vi "Flat Field Estimation.vi"() -> ()   [LabVIEW 2018]
doc: "This example illustrates flat field estimation algorithm. This algorithm estimates the flat field image by surface fitting the background region of the image. Flat field estimation follows two step process. It calculates the background image by using local thresholding methods or surface fitting mathematical model. Once the background image is calculated, surface fit is applied on background image to estimate the flat field image."
uses:
  <vilib>/vision/Process.llb/Background Estimation Options.ctl
  <vilib>/vision/Process.llb/Surface Fit Options.ctl
  <vilib>/vision/NI_Vision_Development_Module.lvlib
panel:
  in  "path":path
  in  "Show Estimated Image?":bool
  in  "Stop":bool
  out "Histograph":T1(graph)
  out "Corrected/Estimated Image":T2(plugin-control)
  out "Part Image":T2(plugin-control)
  in  "Select Image":i32(slide) min=0 max=5 step=1 scale=0.0..3.0
  # "Overview: Demonstrates how to use IMAQ Estimate Flat Field Model to estimate the flat filed image and correct the non uniform intensity using IMAQ Flat Field Correction.\nInstructions:\n1. Run the VI.\n2. Choose images using Select Image control.\n3. Observe the Histograph to understand the impact of correction.\n4. Enable Show Estimated Image boolean to display the estimated flat filed image."
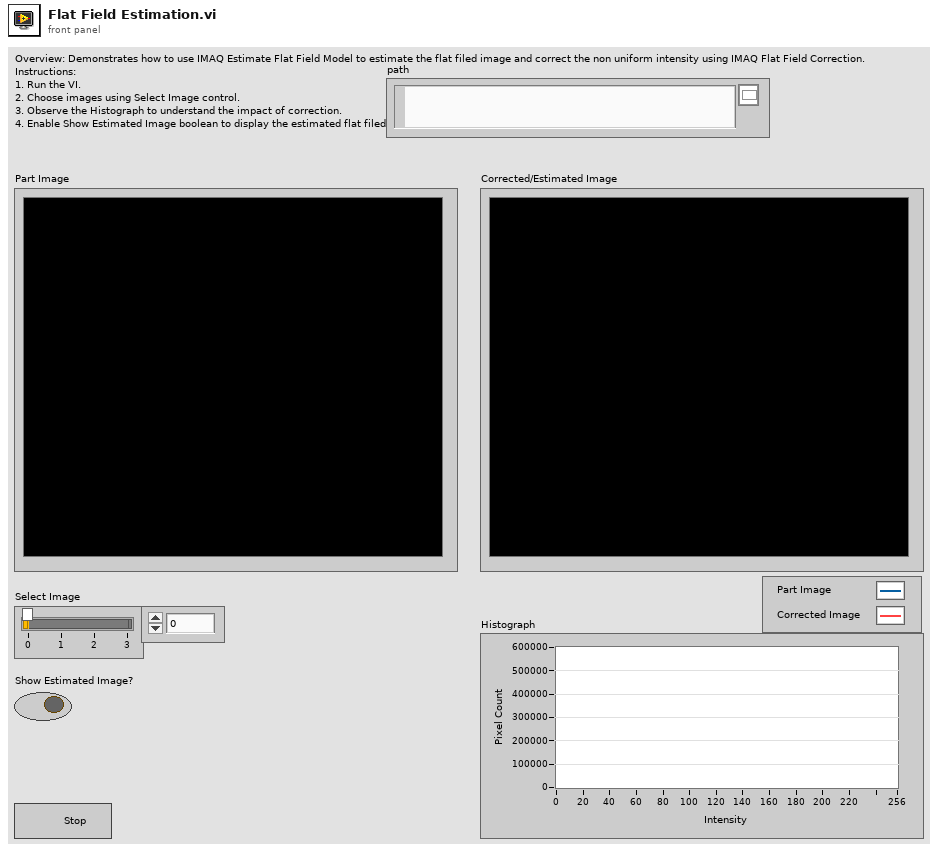
[diagram p1: front panel]
types:
  T1 = cluster{"Starting Value":sgl, "Incremental Value":sgl, "Histogram":u32[]}[]
  T2 = typedef "IMAQ Image.ctl" = refnum<image>
  T3 = typedef "Image Type" = u32
  T4 = cluster{"Line Scan Image?":bool, "Correction Factor":sgl}
  T5 = typedef "Surface Fit Options.ctl" = cluster{"Model":i32, "Sampling Grid Size":cluster{"SizeX":i32, "SizeY":i32}, "Polynomial Degree":i32}
  T6 = typedef "Background Estimation Options.ctl" = cluster{"Estimate Background?":bool, "Method":i32, "Polynomial Degree":i32, "Window Size (32x32)":cluster{"SizeX":i32, "SizeY":i32}, "Niblack Deviation Factor (0.2)":dbl}
  T7 = cluster{"Starting Value":sgl, "Incremental Value":sgl, "Histogram":u32[]}
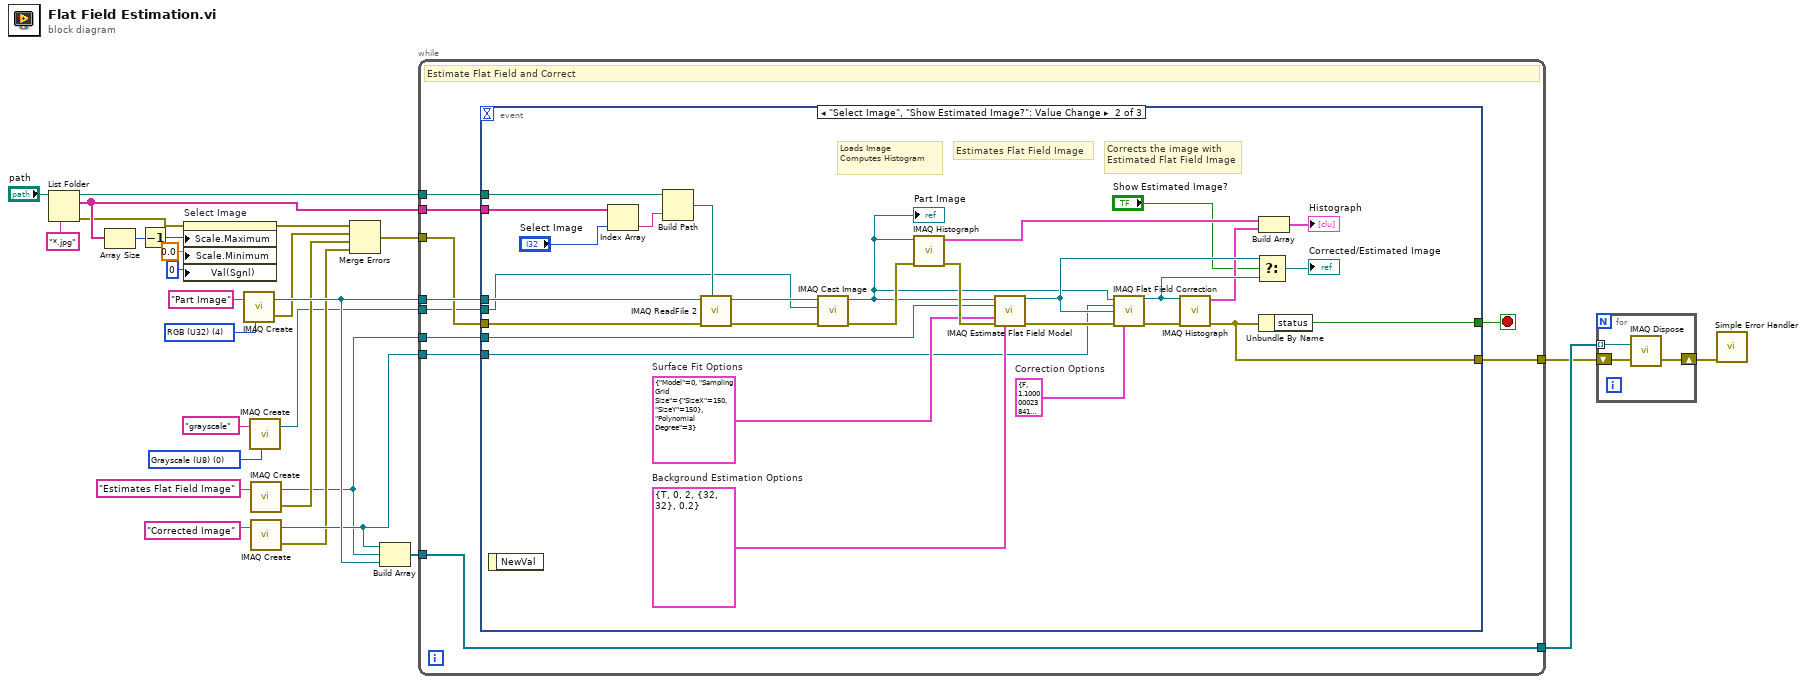
[diagram p0: block diagram]
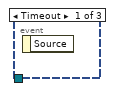
[diagram p2: hidden frame]
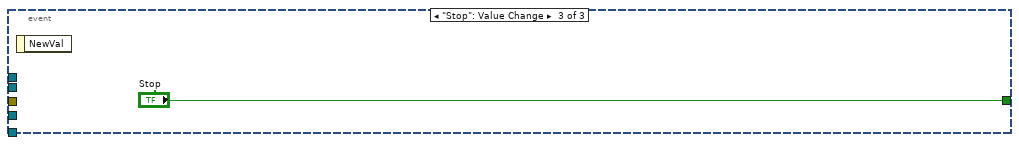
[diagram p3: hidden frame]
diagram:
  w1 = T3 0 items=["Grayscale (U8)", "Grayscale (I16)", "Grayscale (SGL)", "Complex (CSG)", "RGB (U32)", "HSL (U32)", "RGB (U64)", "Grayscale (U16)"] ("Image Type")
  w4 = T3 4 items=["Grayscale (U8)", "Grayscale (I16)", "Grayscale (SGL)", "Complex (CSG)", "RGB (U32)", "HSL (U32)", "RGB (U64)", "Grayscale (U16)"] ("Image Type")
  n1 = List Folder(path="path", pattern="*.jpg") -> (path out=w27:path, filenames=w28:string[], error out=w12:errorcluster)  [unwired: 1 in, 2 out]
  n2 = Array Size(array=w28) -> (size(s)=w24:i32)
  n3 = Decrement(x=w24) -> (x-1=w23:i32)
  n4 = property on="Select Image" class="Slide (strict)"(error in=w12, "Scale.Maximum"=w23, "Scale.Minimum"=0.0 ("Scale.Range:Minimum"), "Val(Sgnl)"=0 ("Value (Signaling)")) -> (error out=w11:errorcluster)  [unwired: 1 in, 1 out]
  n5 = call "IMAQ Create"("Image Name"="Part Image", "Image Type"=w4) -> ("New Image"=w19:T2, "error out"=w17:errorcluster)  [unwired: 3 in]
  n6 = call "IMAQ Create"("Image Name"="grayscale", "Image Type"=w1) -> ("New Image"=w2:T2)  [unwired: 3 in, 1 out]
  n7 = call "IMAQ Create"("Image Name"="Estimates Flat Field Image") -> ("New Image"=w14:T2, "error out"=w16:errorcluster)  [unwired: 4 in]
  n8 = call "IMAQ Create"("Image Name"="Corrected Image") -> ("New Image"=w18:T2, "error out"=w15:errorcluster)  [unwired: 4 in]
  n9 = Merge Errors(w11, w17, w16, w15) -> (w8:errorcluster)
  n10 = Build Array(w18, w14, w19) -> (w10:T2[])
  n11 = while {
    tunnel: w28 -> [w33]
    tunnel: w27 -> [w34]
    tunnel: w19 -> [w38]
    tunnel: w18 -> [w36]
    tunnel: w14 -> [w37]
    tunnel: [w32] -> w9
    tunnel: w10 -> [w32]
    tunnel: w8 -> [w31]
    tunnel: [w30] -> w6
    tunnel: w2 -> [w29]
    stop <- w35 stop-if-true
    # "Estimate Flat Field and Correct"
    n12 = event shown="[1] \"Select Image\", \"Show Estimated Image?\": Value Change" {
      selector: _ -> [_ _ _]
      dyn-events: _ -> [_ _ _]
      timeout: _ -> [_ _ _]
      tunnel: w38 -> [_ w43 _]
      tunnel: w37 -> [_ w53 _]
      tunnel: w36 -> [_ w52 _]
      tunnel: [_ w51 "Stop"] -> w35
      tunnel: w34 -> [_ w50 _]
      tunnel: w33 -> [_ w49 _]
      tunnel: w31 -> [_ w45 _]
      tunnel: [_ w44 _] -> w30
      tunnel: w29 -> [_ w39 _]
      event Timeout {
        n13 = event-data() -> ()  [unwired: 1 in, 1 out]
      }
      event "Select Image", "Show Estimated Image?": Value Change {
        w60 = T4 {"Line Scan Image?"=FALSE, "Correction Factor"=1.1}  # Correction Options
        w54 = T5 {"Model"=0, "Sampling Grid Size"={"SizeX"=150, "SizeY"=150}, "Polynomial Degree"=3}  # Surface Fit Options
        w55 = T6 {"Estimate Background?"=TRUE, "Method"=0, "Polynomial Degree"=2, "Window Size (32x32)"={"SizeX"=32, "SizeY"=32}, "Niblack Deviation Factor (0.2)"=0.2}  # Background Estimation Options
        # "Corrects the image with \nEstimated Flat Field Image"
        # "Estimates Flat Field Image"
        # "Loads Image \nComputes Histogram"
        n14 = event-data() -> ()  [unwired: 1 in, 1 out]
        n15 = Index Array(array=w49, index="Select Image") -> (element=w47:string)
        n16 = Build Path(base path=w50, name or relative path=w47) -> (appended path=w46:path)
        n17 = call "IMAQ ReadFile 2"("File Path"=w46, "error in (no error)"=w45, "Image"=w43) -> ("error out"=w56:errorcluster, "Image Out"=w41:T2)  [unwired: 4 in, 3 out]
        n18 = call "IMAQ Cast Image"("error in (no error)"=w56, "Image Dst"=w39, "Image Src"=w41) -> ("error out"=w42:errorcluster, "Image Dst Out"=w40:T2)  [unwired: 7 in]
        "Part Image" <- w40
        n19 = call "IMAQ Histograph"("error in (no error)"=w42, "Image"=w40) -> ("error out"=w57:errorcluster, "Histogram Graph"=w64:T7)  [unwired: 6 in, 2 out]
        n20 = call "IMAQ Estimate Flat Field Model"("Image Src"=w40, "Image Dst"=w53, "Surface Fit Options"=w54, "error in (no error)"=w57, "Background Estimation Options"=w55) -> ("Flat Field Image Out"=w66:T2, "error out"=w58:errorcluster)  [unwired: 9 in]
        n21 = call "IMAQ Flat Field Correction"("Image Src"=w40, "Image Dst"=w52, "Flat Field Image"=w66, "error in (no error)"=w58, "Correction Options"=w60) -> ("Corrected Image"=w67:T2, "error out"=w59:errorcluster)  [unwired: 8 in, 1 out]
        n22 = call "IMAQ Histograph"("error in (no error)"=w59, "Image"=w67) -> ("error out"=w44:errorcluster, "Histogram Graph"=w63:T7)  [unwired: 6 in, 2 out]
        n23 = Select(t=w66, s="Show Estimated Image?", f=w67) -> (s? t:f=→"Corrected/Estimated Image":T2)
        n24 = Build Array(w64, w63) -> (→"Histograph":T1)
        n25 = Unbundle By Name(w44) -> ("status"=w51:bool)
      }
      event "Stop": Value Change {
        n26 = event-data() -> ()  [unwired: 1 in, 1 out]
      }
    }
  }
  n27 = for {
    tunnel: w9 -> [w71] mode=indexing
    shift-right: [w70] -> w13
    shift-left: w6 -> [w69]
    n28 = call "IMAQ Dispose"("Image"=w71, "error in (no error)"=w69) -> ("error out"=w70:errorcluster)  [unwired: 4 in]
  }
  n29 = call <vilib>:"Simple Error Handler.vi"("error in (no error)"=w13) -> ()  [unwired: 4 in, 5 out]
